vi "Sum_N_factorial.vi"(11 "Input: N":u32) -> (3 "Sum_factorial":i32)   [LabVIEW 2014]
panel:
  # "Sum of factorials till N.\nPlease enter N:"
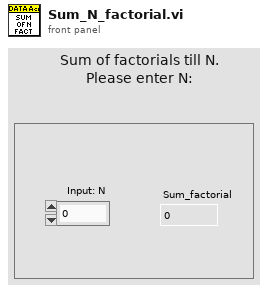
[diagram p1: front panel]
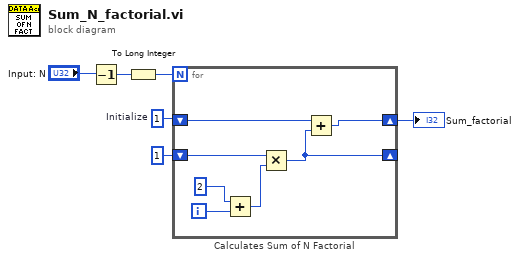
[diagram p0: block diagram]
diagram:
  w5 = 1  # Initialize
  n1 = Decrement(x="Input: N") -> (x-1=w2:u32)
  n2 = To Long Integer(number=w2) -> (32bit integer=w1:i32)
  n3 = for "Calculates Sum of N Factorial" {
    N: w1 -> [_]
    shift-right: [w12] -> _
    shift-left: 1 -> [w11]
    shift-right: [w10] -> w4
    shift-left: w5 -> [w9]
    i -> [w8]
    n4 = Add(x=2 ("y"), y=w8) -> (x+y=w13:i32)
    n5 = Multiply(x=w11, y=w13) -> (x*y=w12:i32)
    n6 = Add(x=w9, y=w12) -> (x+y=w10:i32)
  }
  "Sum_factorial" <- w4
